vi "RH_FGEN_Initialize.vi"(8 "error in":errorcluster, 10 "Simulated HW?":bool, 11 "Resource Name":refnum<k15> caption="FGEN Resource Name") -> (0 "error out":errorcluster, 3 "FGEN Session Out":refnum<k15>)   [LabVIEW 2023, in "ResourceHandling.lvlib"]
doc: "Initialize FGEN resource"
uses:
  ResourceHandling.lvlib
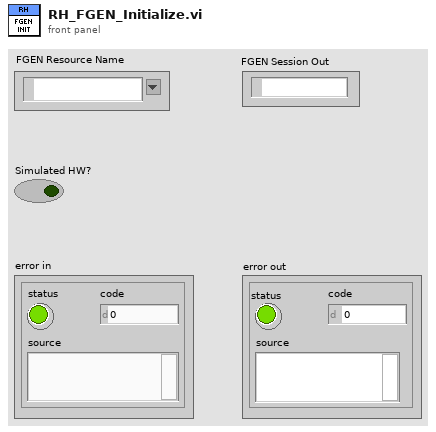
[diagram p1: front panel]
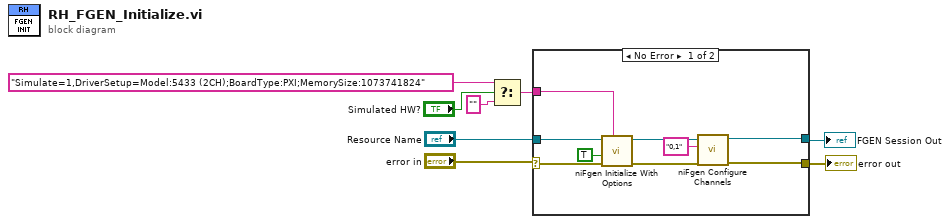
[diagram p0: block diagram]
diagram:
  n1 = Select(t="Simulate=1,DriverSetup=Model:5433 (2CH);BoardType:PXI;MemorySize:1073741824" ("Option String"), s="Simulated HW?", f="") -> (s? t:f=w6:string)
  n2 = case shown="No Error" "error in" {
    selector: "error in" -> [w15 w19]
    tunnel: w6 -> [w17 _]
    tunnel: [w11 w19] -> w5
    tunnel: "Resource Name" -> [w16 w18]
    tunnel: [w10 w18] -> w1
    frame No Error {
      n3 = call <instrlib>:"niFgen Initialize With Options.vi"("Option String"=w17, "error in (no error)"=w15, "Reset Device (default: True)"=TRUE, "Resource Name"=w16) -> ("error out"=w13:errorcluster, "Instrument Handle Out"=w12:refnum<k15>)  [unwired: 6 in]
      n4 = call <instrlib>:"niFgen Configure Channels.vi"("error in (no error)"=w13, "Channels"="0,1", "Instrument Handle"=w12) -> ("error out"=w11:errorcluster, "Instrument Handle Out"=w10:refnum<k15>)  [unwired: 7 in]
    }
    frame Error {
    }
  }
  "error out" <- w5
  "FGEN Session Out" <- w1
